vi "VISA(Write).vi"(8 "error in (no error)":errorcluster caption="错误输入（无错误）", 10 "写入缓冲区":string, 11 "VISA资源名称":refnum<visa-resource-name>) -> (0 "error out":errorcluster caption="错误输出", 3 "VISA资源名称输出":refnum<visa-resource-name>)   [LabVIEW 2020, in "人体健康监测系统.lvclass"]
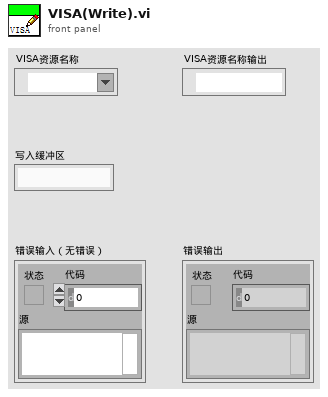
[diagram p1: front panel]
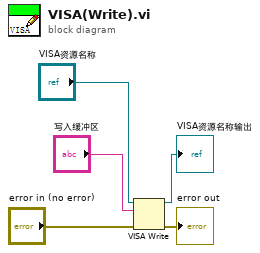
[diagram p0: block diagram]
diagram:
  n1 = VISA Write(VISA resource name="VISA资源名称", write buffer="写入缓冲区", error in (no error)="error in (no error)") -> (VISA resource name out=→"VISA资源名称输出":refnum<visa-resource-name>, error out=→"error out":errorcluster)  [unwired: 1 out]
